vi "Filter-and-storage-wrapper.vi"(8 "error in":errorcluster, 11 "Data ref. in":refnum<data-value>) -> (0 "error IO":errorcluster, 3 "Data ref.":refnum<data-value>)   [LabVIEW 2013, in "CameraVision.lvlib" / "CV-Main.lvclass"]
uses:
  CV-Main.lvclass
  CV-Main.lvclass/CV-Main.ctl
  Buffers/CV-Buffers.lvclass/CV-Buffers.ctl
  Filter/CV-Filter.lvclass/CV-Filter.ctl
  UI/Module-states.ctl
  UI/Notifier-with-memory-boolean.vi
  Read Filter params.vi
  Read Storage params.vi
  Read Processing.vi
  Read Buffers.vi
  Buffers/Read Storage buffer.vi
  Filter/Read Filter array temp.vi
  Filter/CV-Filter.lvclass
  Storage/CV-Storage.lvclass
  Buffers/CV-Buffers.lvclass
  UI/CV-UI.lvclass
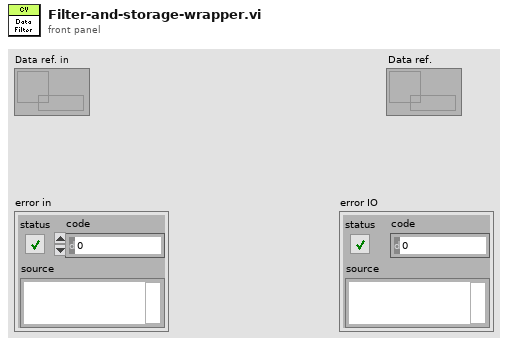
[diagram p1: front panel]
types:
  T1 = typedef "CameraVision.lvlib/CV-UI.lvclass/Module-states.ctl" = enum16{"Inactive", "Active", "Data-loss", "Error", "Simulation", "Synchronizing", "Initialized", "Released"}
  T2 = typedef "CameraVision.lvlib/Filter.lvclass/Filter-settings.ctl" = cluster{"Characteristic":T3, "Monitor":bool, "Min.":dbl, "Max.":dbl, "Min. Thres.":dbl, "Min. Dur.":u16, "Report":bool}
  T3 = typedef "CameraVision.lvlib/Filter.lvclass/Filter-characteristic.ctl" = enum16{"Average intensity [0-255]", "Peak intensity [0-255]", "Melt-pool size [mm²]", "Melt-pool aspect ratio []", "Melt-pool fragments []", "Melt-pool position X [pixel]", "Melt-pool position Y [pixel]", "Average temperature [°C]", "Max. temperature [°C]", "Min. temperature [°C]", "Std. dev. temperature [°C]"}
  T4 = typedef "CameraVision.lvlib/Buffers.lvclass/Storage-buffer.ctl" = cluster{"Index":i32, "Time":timestamp, "Raw images":T5[], "Corrected images":T5[], "Binary images":T5[], "Temperature characteristics":T6, "Characteristics":T7[], "Temperature field":dbl[][]}
  T5 = typedef "IMAQ Image.ctl" = refnum<image>
  T6 = typedef "CameraVision.lvlib/Temperature.lvclass/Temperature-characteristics.ctl" = cluster{"Average temperature ":dbl, "Max. temperature":dbl, "Min. temperature":dbl, "Stand. dev. temperature":dbl, "Datapoints":dbl}
  T7 = typedef "CameraVision.lvlib/Analysis.lvclass/Characteristics-cluster.ctl" = cluster{"Average intensity":dbl, "Peak intensity":dbl, "Melt-pool size":dbl, "Melt-pool aspect ratio":dbl, "Melt-pool fragments":dbl, "Centre of mass X":dbl, "Centre of mass Y":dbl, "Orientation":dbl}
  T8 = typedef "CameraVision.lvlib/CV-Buffers.lvclass/Storage-buffer.ctl" = cluster{"Index":i32, "Time":timestamp, "Raw images":T5[], "Corrected images":T5[], "Binary images":T5[], "Temperature characteristics":T9, "Characteristics":T10[], "Temperature field":dbl[][]}
  T9 = typedef "CameraVision.lvlib/CV-Temperature.lvclass/Temperature-characteristics.ctl" = cluster{"Average temperature ":dbl, "Max. temperature":dbl, "Min. temperature":dbl, "Stand. dev. temperature":dbl, "Datapoints":dbl}
  T10 = typedef "CameraVision.lvlib/CV-Analysis.lvclass/Characteristics-cluster.ctl" = cluster{"Average intensity":dbl, "Peak intensity":dbl, "Melt-pool size":dbl, "Melt-pool aspect ratio":dbl, "Melt-pool fragments":dbl, "Centre of mass X":dbl, "Centre of mass Y":dbl, "Orientation":dbl}
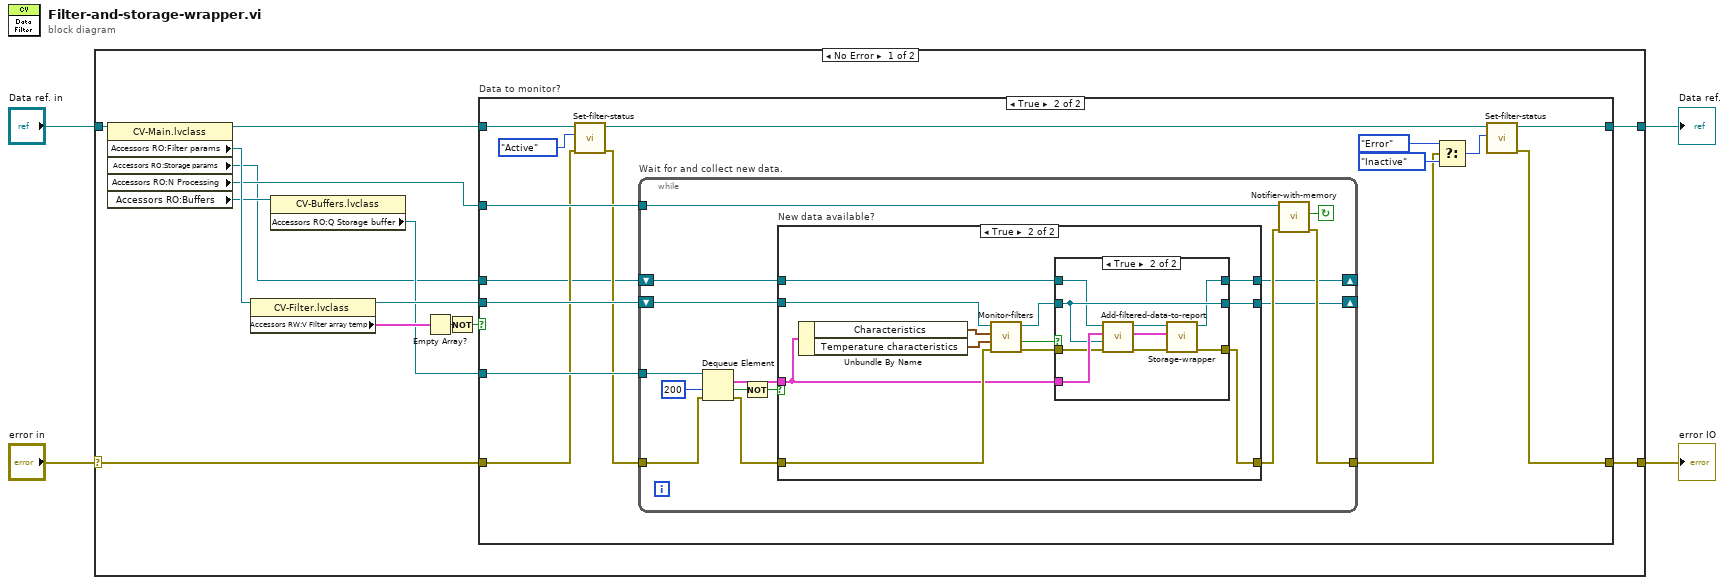
[diagram p0: block diagram]
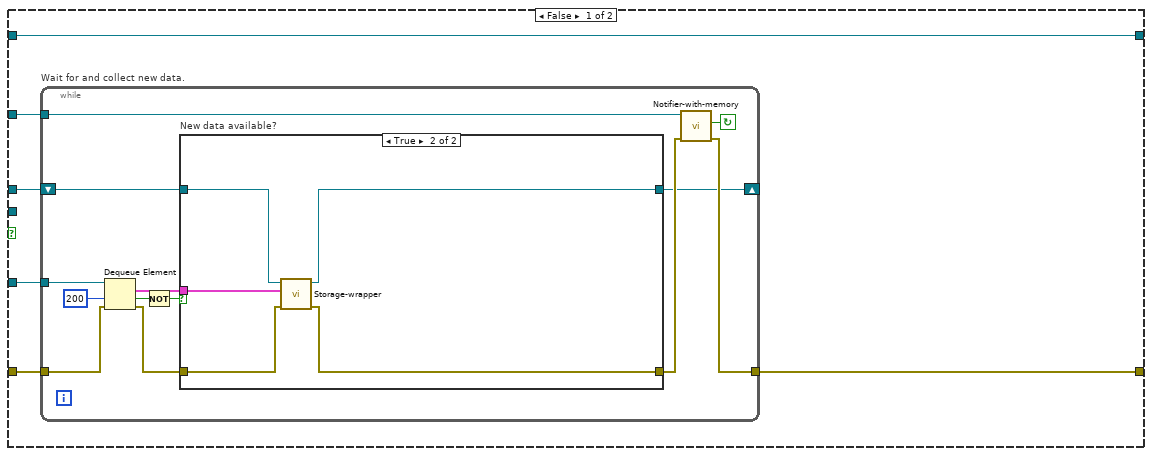
[diagram p2: hidden frame]
diagram:
  n1 = case shown="No Error" "error in" {
    selector: "error in" -> [w12 w103]
    tunnel: [w5 w103] -> w4
    tunnel: "Data ref. in" -> [w14 w102]
    tunnel: [w6 w102] -> w1
    frame No Error {
      n2 = property class="CV-Main.lvclass"(reference=w14) -> (reference out=w11:refnum<data-value>, "Accessors RO:Filter params"=w13:refnum<data-value>, "Accessors RO:Storage params"=w7:refnum<data-value>, "Accessors RO:N Processing"=w10:refnum<notifier>, "Accessors RO:Buffers"=w9:refnum<class "CV-Buffers.lvclass">)  [unwired: 1 in, 1 out]
      n3 = property class="CV-Filter.lvclass"(reference=w13) -> (reference out=w15:refnum<data-value>, "Accessors RW:V Filter array temp"=w18:T2[])  [unwired: 1 in, 1 out]
      n4 = property class="CV-Buffers.lvclass"(reference=w9) -> ("Accessors RO:Q Storage buffer"=w8:refnum<queue>)  [unwired: 1 in, 2 out]
      n5 = Empty Array?(array=w18) -> (empty?=w17:bool)
      n6 = Not(x=w17) -> (.not. x?=w16:bool)
      n7 = case "Data to monitor?" shown="True" w16 {
        tunnel: [w19 w45] -> w5
        tunnel: w10 -> [w24 w59]
        tunnel: w15 -> [_ w58]
        tunnel: w12 -> [w21 w51]
        tunnel: w11 -> [w20 w57]
        tunnel: [w20 w46] -> w6
        tunnel: w8 -> [w22 w55]
        tunnel: w7 -> [w23 w47]
        frame False {
          n8 = while "Wait for and collect new data." {
            tunnel: [w35] -> w19
            tunnel: w24 -> [w37]
            tunnel: w22 -> [w33]
            shift-right: [w26] -> _
            shift-left: w23 -> [w27]
            tunnel: w21 -> [w25]
            stop <- w36 continue-if-true
            n9 = Dequeue Element(queue=w33, timeout in ms (-1)=200, error in (no error)=w25) -> (element=w31:T4, timed out?=w30:bool, error out=w28:errorcluster)  [unwired: 1 out]
            n10 = Not(x=w30) -> (.not. x?=w29:bool)
            n11 = case "New data available?" shown="True" w29 {
              tunnel: [w39 w40] -> w34
              tunnel: w28 -> [w39 w41]
              tunnel: w31 -> [_ w43]
              tunnel: w27 -> [w38 w44]
              tunnel: [w38 w42] -> w26
              frame False {
              }
              frame True {
                n12 = call "Storage-wrapper.vi"("error in"=w41, "Storage element in"=w43, "Storage params. ref. in"=w44) -> ("error IO"=w40:errorcluster, "Storage params. ref."=w42:refnum<data-value>)  [unwired: 6 in, 1 out]
              }
            }
            n13 = call-poly "Notifier-with-memory.vi"("error in"=w34, "Notifier in"=w37) -> ("error IO"=w35:errorcluster, "Notification"=w36:bool)  [unwired: 8 in]
          }
        }
        frame True {
          n14 = call "Set-filter-status.vi"("error in"=w51, "Filter status in"=Module-states."Active" ("Filter status"), "Data ref. in"=w57) -> ("error IO"=w50:errorcluster, "Data ref."=w49:refnum<data-value>)  [unwired: 6 in, 1 out]
          n15 = while "Wait for and collect new data." {
            tunnel: [w72] -> w48
            tunnel: w50 -> [w63]
            tunnel: w59 -> [w74]
            shift-right: [w69] -> _
            shift-left: w58 -> [w70]
            tunnel: w55 -> [w68]
            shift-right: [w60] -> _
            shift-left: w47 -> [w61]
            stop <- w73 continue-if-true
            n16 = Dequeue Element(queue=w68, timeout in ms (-1)=200, error in (no error)=w63) -> (element=w66:T4, timed out?=w65:bool, error out=w62:errorcluster)  [unwired: 1 out]
            n17 = Not(x=w65) -> (.not. x?=w64:bool)
            n18 = case "New data available?" shown="True" w64 {
              tunnel: [w77 w78] -> w71
              tunnel: w62 -> [w77 w88]
              tunnel: w70 -> [w76 w89]
              tunnel: [w76 w81] -> w69
              tunnel: w66 -> [_ w80]
              tunnel: w61 -> [w75 w83]
              tunnel: [w75 w82] -> w60
              frame False {
              }
              frame True {
                n19 = Unbundle By Name(w80) -> ("Characteristics"=w87:T7[], "Temperature characteristics"=w86:T6)
                n20 = call "Monitor-filters.vi"("error in"=w88, "Temperature characteristics"=w86, "Characteristics"=w87, "Filter params. ref. in"=w89) -> ("error IO"=w79:errorcluster, "Add to report?"=w85:bool, "Filter params. ref."=w84:refnum<data-value>)  [unwired: 5 in]
                n21 = case shown="True" w85 {
                  tunnel: w84 -> [w91 w99]
                  tunnel: w83 -> [w92 w97]
                  tunnel: [w92 w96] -> w82
                  tunnel: [w91 w99] -> w81
                  tunnel: w80 -> [_ w100]
                  tunnel: w79 -> [w90 w94]
                  tunnel: [w90 w93] -> w78
                  frame False {
                  }
                  frame True {
                    n22 = call "Add-filtered-data-to-report.vi"("error in"=w94, "Filter params. ref. in"=w99, "Storage element in"=w100, "Storage params. ref. in"=w97) -> ("error IO"=w101:errorcluster, "Storage element"=w95:T8, "Storage params. ref."=w98:refnum<data-value>)  [unwired: 4 in, 1 out]
                    n23 = call "Storage-wrapper.vi"("error in"=w101, "Storage element in"=w95, "Storage params. ref. in"=w98) -> ("error IO"=w93:errorcluster, "Storage params. ref."=w96:refnum<data-value>)  [unwired: 6 in, 1 out]
                  }
                }
              }
            }
            n24 = call-poly "Notifier-with-memory.vi"("error in"=w71, "Notifier in"=w74) -> ("error IO"=w72:errorcluster, "Notification"=w73:bool)  [unwired: 8 in]
          }
          n25 = Select(t=Module-states."Error" ("Filter status"), s=w48, f=Module-states."Inactive") -> (s? t:f=w54:T1)
          n26 = call "Set-filter-status.vi"("Filter status in"=w54, "Data ref. in"=w49) -> ("error IO"=w45:errorcluster, "Data ref."=w46:refnum<data-value>)  [unwired: 7 in, 1 out]
        }
      }
    }
    frame Error {
    }
  }
  "error IO" <- w4
  "Data ref." <- w1
